vi "Close.vi"(8 "error in (no error)":errorcluster, 11 "Logger in":refnum<class "Logger.lvclass">) -> (0 "error out":errorcluster)   [LabVIEW 2013, in "Logger.lvclass"]
doc: "Properly closes a Logger Object.\n\n<b>It is critical that all initialized Logger objects are closed with the Close method.</b> This method signals the background process to stop. If the Close method is not called, the background process will continue to run on the host computer. For this reason, <b>do not abort an application which uses Logger Objects.</b>\n\nJared Kirschner, 2012."
uses:
  Logger.lvclass
  Logger.lvclass/Logger.ctl
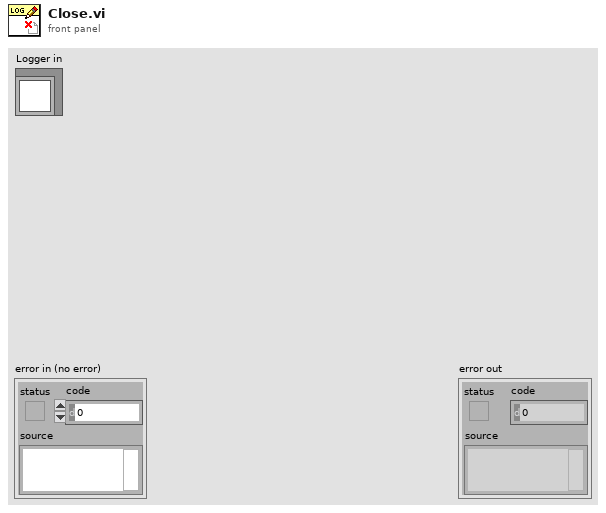
[diagram p1: front panel]
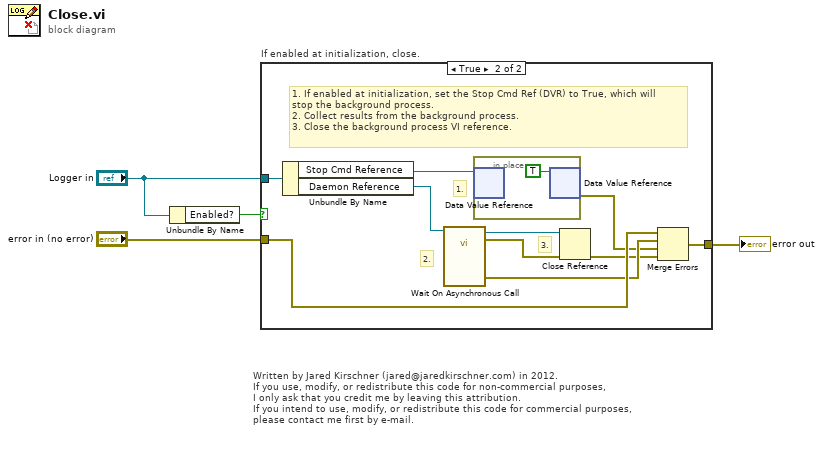
[diagram p0: block diagram]
diagram:
  # "Written by Jared Kirschner (jared@jaredkirschner.com) in 2012.\nIf you use, modify, or redistribute this code for non-commercial purposes,\nI only ask that you credit me by leaving this attribution.\nIf you intend to use, modify, or redistribute this code for commercial purposes,\nplease contact me first by e-mail."
  n1 = Unbundle By Name("Logger in") -> ("Enabled?"=w1:bool)
  n2 = case "If enabled at initialization, close." shown="True" w1 {
    tunnel: "Logger in" -> [_ w15]
    tunnel: [w5 w13] -> w4
    tunnel: "error in (no error)" -> [w5 w9]
    frame False {
      # "If not enabled at initialization, do nothing,\nas there are no resources to close!"
    }
    frame True {
      # "3."
      # "2."
      # "1."
      # "1. If enabled at initialization, set the Stop Cmd Ref (DVR) to True, which will\nstop the background process.\n2. Collect results from the background process.\n3. Close the background process VI reference."
      n3 = Unbundle By Name(w15) -> ("Stop Cmd Reference"=w14:refnum<data-value>, "Daemon Reference"=w12:refnum<vi>)
      n4 = call-by-ref "Wait On Asynchronous Call"(reference=w12) -> (reference out=w11:refnum<vi>, error out=w10:errorcluster, 0:"error out"=w8:errorcluster)  [unwired: 12 in]
      n5 = in-place {
        n6 = in-place-dvr #1(w14) -> ()  [unwired: 2 out]
        n7 = in-place-dvr #1(TRUE ("data value")) -> (w7:errorcluster)  [unwired: 1 out]
      }
      n8 = Close Reference(reference=w11, error in (no error)=w10) -> (error out=w6:errorcluster)
      n9 = Merge Errors(w9, w8, w7, w6) -> (w13:errorcluster)
    }
  }
  "error out" <- w4
